vi "Convert Array to Image (SubVI).vi"(5 "Image Size":T1={"Height"=512, "Width"=512} {"Width" step=8; "Height" step=8}, 11 "Image Array In":u64[](array[numeric])) -> (2 "Image Array Out":u8[][](array[numeric]))   [LabVIEW 2020]
uses:
  Controls (HOST)/Image Size.ctl
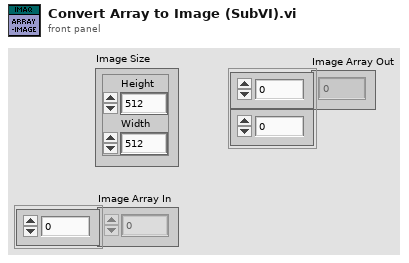
[diagram p1: front panel]
types:
  T1 = typedef "Image Size.ctl" = cluster{"Height":u16, "Width":u16}
  T2 = enum16{"big-endian, network order", "native, host order", "little-endian"}
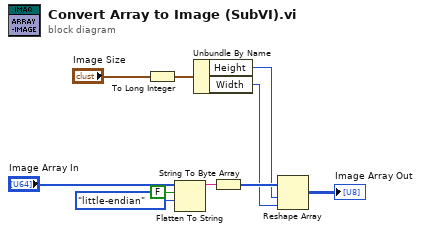
[diagram p0: block diagram]
diagram:
  n1 = To Long Integer(number="Image Size") -> (32bit integer=w9:cluster{"Height":i32, "Width":i32})
  n2 = Flatten To String(anything="Image Array In", prepend array or string size? (T)=FALSE, byte order (0:big-endian, network order)=T2."little-endian") -> (data string=w6:string)  [unwired: 1 in, 2 out]
  n3 = Unbundle By Name(w9) -> ("Height"=w3:i32, "Width"=w2:i32)
  n4 = String To Byte Array(string=w6) -> (unsigned byte array=w5:u8[])
  n5 = Reshape Array(w5, w3, w2) -> (→"Image Array Out":u8[][])
